vi "Peregrine_init.vi"(5 "COM Port for serial\nconnection. Check device\nmanager.":string) -> (0 "error out":errorcluster, 2 "Handle out":refnum<visa-resource-name>)   [LabVIEW 2019]
uses:
  <vilib>/Instr/_visa.llb/VISA Configure Serial Port (Instr).vi
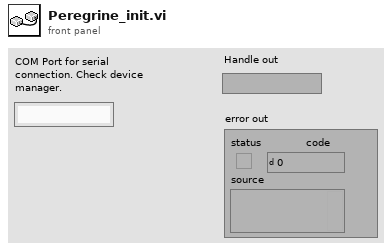
[diagram p1: front panel]
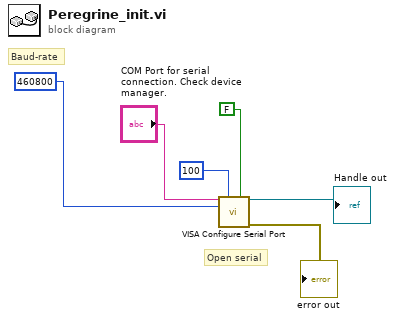
[diagram p0: block diagram]
diagram:
  # "Open serial"
  # "Baud-rate"
  n1 = call-poly "VISA Configure Serial Port"("VISA resource name"="COM Port for serial\nconnection. Check device\nmanager.", "timeout (10sec)"=u32 100, "Enable Termination\nChar (T)"=FALSE ("Enable Termination\nChar (T)"), "baud rate (9600)"=460800) -> ("VISA resource name out"=→"Handle out":refnum<visa-resource-name>, "error out"=→"error out":errorcluster)  [unwired: 10 in]
